vi "Set NotifyIcon Visibility.vi"(4 "error in (no error)":errorcluster, 6 "Visible":bool, 7 "NotifyIcon in":refnum<k24>) -> (0 "error out":errorcluster, 3 "NotifyIcon out":refnum<k24>)   [LabVIEW 2014, in "NotifyIcon.lvlib"]
uses:
  NotifyIcon.lvlib
  System.Windows.Forms
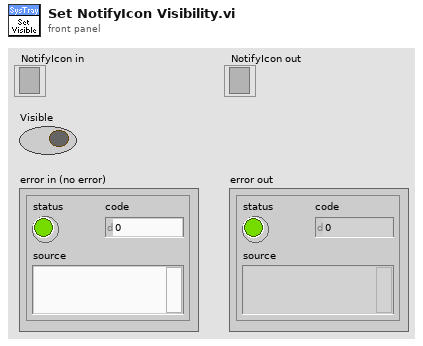
[diagram p1: front panel]
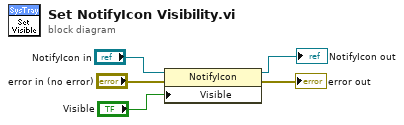
[diagram p0: block diagram]
diagram:
  n1 = property class="NotifyIcon"(reference="NotifyIcon in", error in="error in (no error)", "Visible"="Visible") -> (reference out=→"NotifyIcon out":refnum<k24>, error out=→"error out":errorcluster)
